vi "Check If Done.vi"(8 "error in (no error)":errorcluster, 11 "Motion In":refnum<class "BasicTerminalBinding.lvclass">) -> (0 "error out":errorcluster, 3 "Motion Out":refnum<class "BasicTerminalBinding.lvclass">)   [LabVIEW 2017, in "TestViewables.lvlib" / "BasicTerminalBinding.lvclass"]
uses:
  BasicTerminalBinding.lvclass
  C:/Program Files (x86)/National Instruments/LabVIEW 2017/vi.lib/ActorFramework/Actor/Actor.lvclass
  <vilib>/ActorFramework/Actor/Actor.lvclass/Actor.ctl
  <vilib>/ActorFramework/Message Enqueuer/Message Enqueuer.lvclass/Message Enqueuer.ctl
  <vilib>/ActorFramework/Message Enqueuer/Init from Existing Queue.vi
  <vilib>/ActorFramework/Message Enqueuer/Enqueue.vi
  BasicTerminalBinding Messages/Check If Done Msg/Check If Done Msg.lvclass
  C:/Program Files (x86)/National Instruments/LabVIEW 2017/vi.lib/ActorFramework/Message/Message.lvclass
  <vilib>/ActorFramework/Message Priority Queue/Priority Enqueue.vi
  <vilib>/ActorFramework/Message Enqueuer/Message Enqueuer.lvclass
  <vilib>/ActorFramework/Actor/Actor.lvclass
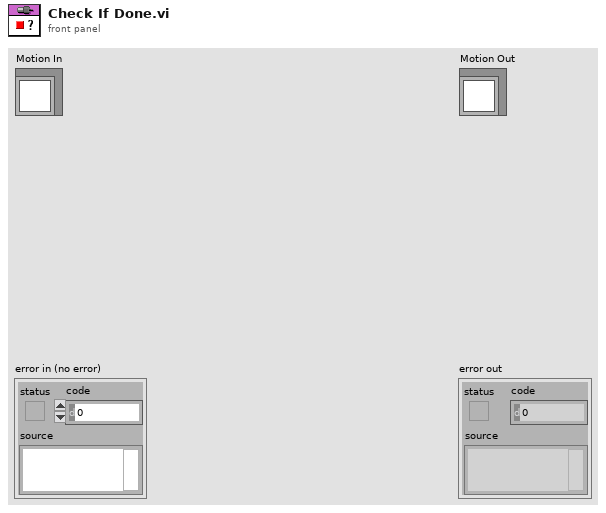
[diagram p1: front panel]
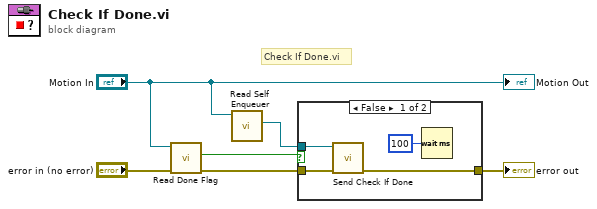
[diagram p0: block diagram]
diagram:
  # "Check If Done.vi"
  n1 = call "Read Done Flag.vi"("error in (no error)"="error in (no error)", "BasicTerminalBinding in"="Motion In") -> ("error out"=w5:errorcluster, "Done?"=w1:bool)  [unwired: 8 in]
  n2 = call <vilib>:"Read Self Enqueuer.vi"("Actor"="Motion In") -> ("Self Enqueuer"=w2:refnum<class "Message Enqueuer.lvclass">)  [unwired: 10 in]
  n3 = case shown="False" w1 {
    tunnel: w5 -> [w10 w11]
    tunnel: [w9 w11] -> w3
    tunnel: w2 -> [w8 _]
    frame False {
      n4 = call "Send Check If Done.vi"("error in (no error)"=w10, "Message Enqueuer"=w8) -> ("error out"=w9:errorcluster)  [unwired: 8 in, 1 out]
      n5 = Wait (ms)(milliseconds to wait=u32 100) -> ()  [unwired: 1 out]
    }
    frame True {
    }
  }
  "error out" <- w3
  "Motion Out" <- "Motion In"
